vi "testaa.vi"() -> ()   [LabVIEW 2020]
panel:
  out "Path":path
  out "pliki":string[](array[string])
  out "error out":errorcluster
  in  "error in (no error) 2":errorcluster
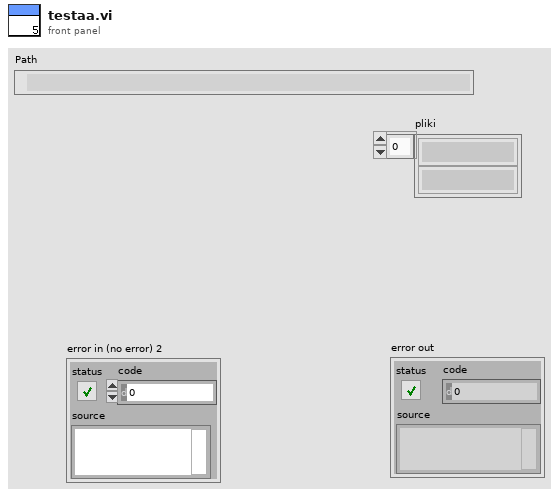
[diagram p1: front panel]
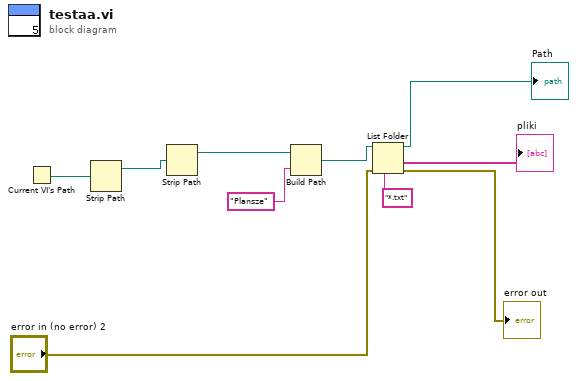
[diagram p0: block diagram]
diagram:
  n1 = Current VI's Path() -> (path=w1:path)
  n2 = Strip Path(path=w1) -> (stripped path=w2:path)  [unwired: 1 out]
  n3 = Strip Path(path=w2) -> (stripped path=w3:path)  [unwired: 1 out]
  n4 = Build Path(base path=w3, name or relative path="Plansze") -> (appended path=w8:path)
  n5 = List Folder(path=w8, pattern="*.txt", error in="error in (no error) 2") -> (path out=→"Path":path, folder names=→"pliki":string[], error out=→"error out":errorcluster)  [unwired: 1 in, 1 out]
